vi "9093_第3回課題_ 山口修平.vi"() -> ()   [LabVIEW 2020]
panel:
  out "現在の回数":dbl
  out "学生番号":dbl
  in  "回数":dbl
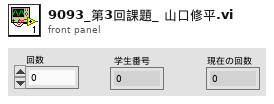
[diagram p1: front panel]
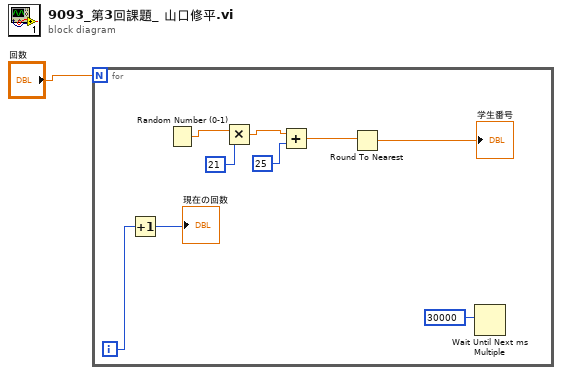
[diagram p0: block diagram]
diagram:
  n1 = for {
    N: "回数" -> [_]
    i -> [w10]
    n2 = Increment(x=w10) -> (x+1=→"現在の回数":i32)
    n3 = Random Number (0-1)() -> (number: 0 to 1=w8:dbl)
    n4 = Multiply(x=w8, y=21) -> (x*y=w7:dbl)
    n5 = Add(x=w7, y=25) -> (x+y=w6:dbl)
    n6 = Round To Nearest(number=w6) -> (nearest integer value=→"学生番号":dbl)
    n7 = Wait Until Next ms Multiple(millisecond multiple=30000) -> ()  [unwired: 1 out]
  }
